vi "gl_Binary time series files globals.vi"() -> ()   [LabVIEW 2017]
panel:
  out "Set2":bool
  out "Set1":bool
  in  "Binary ref 2":refnum<file>
  in  "Binary ref":refnum<file>
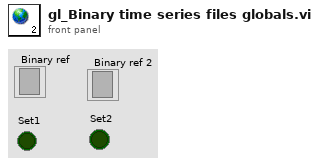
[diagram p1: front panel]
diagram:
